vi "Initialize Data Channels.vi"(8 "error in (no error)":errorcluster, 10 "Framework Configuration":refnum<class "Framework Configuration.lvclass">, 11 "VeriStand Data Sharing Framework in":refnum<class "VeriStand DSF.lvclass">) -> (0 "error out":errorcluster, 1 "data channels refs":T1[](array[typedef]) format="%.0x", 2 "data channel offsets":u64[](array[numeric]) format="%.0x", 3 "VeriStand Data Sharing Framework out":refnum<class "VeriStand DSF.lvclass">)   [LabVIEW 2020, in "DSF Engine.lvlib" / "VeriStand DSF.lvclass"]
uses:
  VeriStand DSF.lvclass
  DSF Core.lvlibp/Classes/Configuration/Core/Framework/Framework Configuration.lvclass
  <vilib>/NI VeriStand/Custom Device API/Custom Device Item Ref.ctl
  VeriStand DSF.lvclass/VeriStand DSF.ctl
  <vilib>/NI VeriStand/Custom Device API/Data Access Type.ctl
  DSF Core.lvlibp/Typedefs/DSF Direction.ctl
  Data Channel Page GUID.vi
  <vilib>/NI VeriStand/Custom Device API/Custom Device API.lvlib
  Source/DSF Core.lvlibp
  DSF Shared.lvlib
  DSF Core.lvlibp/Classes/Configuration/Core/Thread/Thread Configuration.lvclass
  DSF Core.lvlibp/Classes/Configuration/Core/Plugin/Plugin Configuration.lvclass
  DSF Core.lvlibp/Classes/Configuration/Core/Group/Group Configuration.lvclass
  DSF Core.lvlibp/Classes/Configuration/Core/Transfer/Transfer Configuration.lvclass
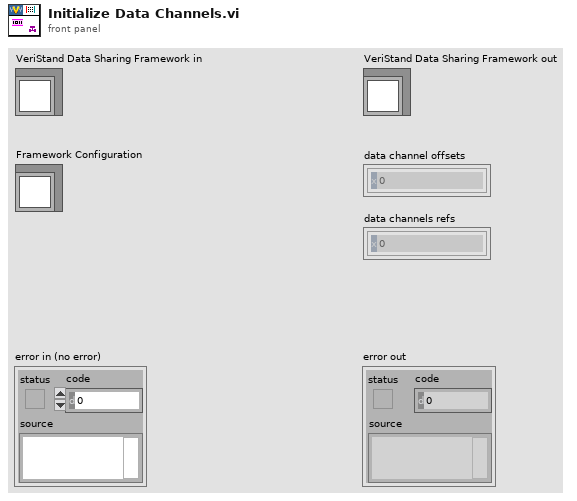
[diagram p1: front panel]
types:
  T1 = typedef "Custom Device API.lvlib/Custom Device Item Ref.ctl" = u64
  T2 = typedef "Custom Device API.lvlib/Data Access Type.ctl" = enum16{"Read", "Write"}
  T3 = typedef "DSF Core.lvlibp/DSF Direction.ctl" = enum8{"Tx", "Rx"}
  T4 = typedef "DSF Core.lvlibp/Group Configuration.lvclass/Core Group Configuration.ctl" = cluster{"name":string, "direction":T3, "cycle timing":T5, "timeout behavior":T6, "enable conversion":bool}
  T5 = typedef "DSF Core.lvlibp/DSF Timing Info.ctl" = cluster{"priority":u64, "decimation":u64, "offset":u64}
  T6 = typedef "DSF Core.lvlibp/DSF Timeout Behavior.ctl" = enum8{"Increment Late Count", "Throw Error"}
  T7 = typedef "DSF Core.lvlibp/Transfer Configuration.lvclass/Channel Configuration.ctl" = cluster{"configuration":T8, "component settings":T10[]}
  T8 = typedef "DSF Core.lvlibp/Channel Configuration.lvclass/Core Channel Configuration.ctl" = cluster{"name":string, "units":string, "engine data type":T9, "string data type":T9, "string offset":u64}
  T9 = typedef "DSF Core.lvlibp/DSF Data Type.ctl" = enum8{"Bool", "SGL", "DBL", "I8", "I16", "I32", "I64", "U8", "U16", "U32", "U64"}
  T10 = typedef "DSF Core.lvlibp/DSF Settings Info.ctl" = cluster{"component":string, "values":cluster{"key":string, "value":string}[]}
  T11 = typedef "Custom Device API.lvlib/Data Reference.ctl" = i32
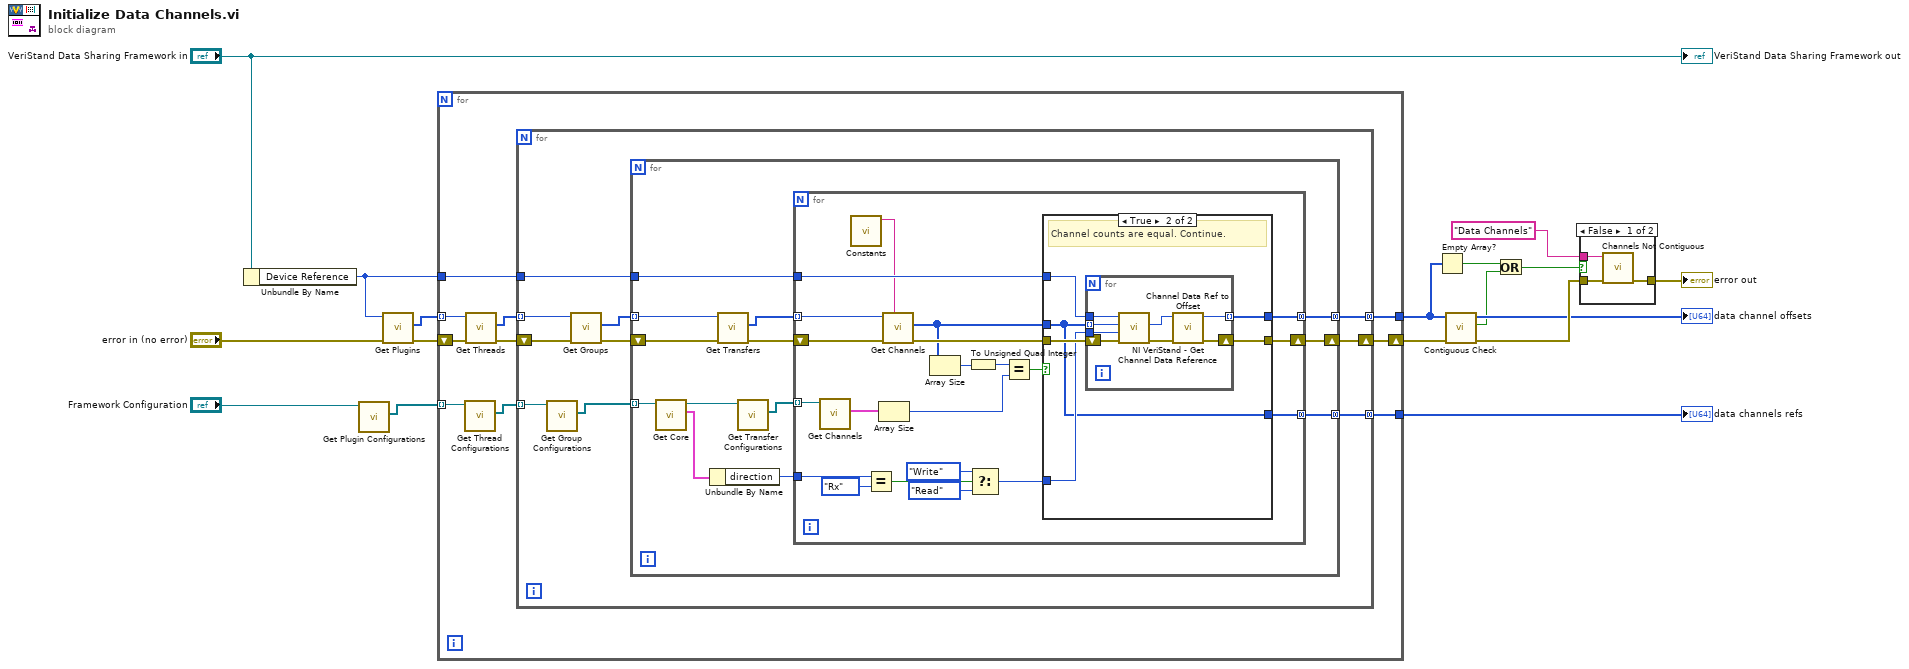
[diagram p0: block diagram]
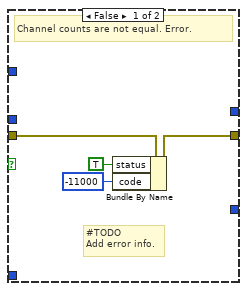
[diagram p2: hidden frame]
diagram:
  n1 = Unbundle By Name("VeriStand Data Sharing Framework in") -> ("Device Reference"=w13:T1)
  n2 = call "Get Plugin Configurations.vi"("Framework Configuration in"="Framework Configuration") -> ("Plugin Configurations"=w3:refnum<class "Plugin Configuration.lvclass">[])  [unwired: 8 in, 2 out]
  n3 = call "Get Plugins.vi"("error in (no error)"="error in (no error)", "Item Ref in"=w13) -> ("error out"=w16:errorcluster, "Plugin refs"=w15:T1[])  [unwired: 7 in, 1 out]
  n4 = for {
    tunnel: w15 -> [w22] mode=indexing
    tunnel: w13 -> [w26]
    tunnel: [w25] -> w10
    tunnel: [w24] -> w9
    tunnel: w3 -> [w19] mode=indexing
    shift-right: [w27] -> w17
    shift-left: w16 -> [w23]
    n5 = call "Get Thread Configurations.vi"("Plugin Configuration in"=w19) -> ("Thread Configurations"=w18:refnum<class "Thread Configuration.lvclass">[])  [unwired: 8 in, 2 out]
    n6 = call "Get Threads.vi"("error in (no error)"=w23, "Item Ref in"=w22) -> ("error out"=w21:errorcluster, "Plugin refs"=w20:T1[])  [unwired: 7 in, 1 out]
    n7 = for {
      tunnel: w20 -> [w33] mode=indexing
      tunnel: w18 -> [w29] mode=indexing
      tunnel: w26 -> [w37]
      shift-right: [w36] -> w27
      shift-left: w21 -> [w34]
      tunnel: [w35] -> w24 mode=concatenating
      tunnel: [w30] -> w25 mode=concatenating
      n8 = call "Get Group Configurations.vi"("Thread Configuration in"=w29) -> ("Group Configurations"=w28:refnum<class "Group Configuration.lvclass">[])  [unwired: 8 in, 2 out]
      n9 = call "Get Groups.vi"("error in (no error)"=w34, "Plugin Ref in"=w33) -> ("error out"=w32:errorcluster, "Group refs"=w31:T1[])  [unwired: 7 in, 1 out]
      n10 = for {
        tunnel: w28 -> [w42] mode=indexing
        tunnel: w31 -> [w46] mode=indexing
        tunnel: w37 -> [w50]
        shift-right: [w49] -> w36
        shift-left: w32 -> [w47]
        tunnel: [w48] -> w35 mode=concatenating
        tunnel: [w43] -> w30 mode=concatenating
        n11 = call "Get Core.vi"("Group Configuration in"=w42) -> ("core"=w38:T4, "Group Configuration out"=w41:refnum<class "Group Configuration.lvclass">)  [unwired: 8 in, 1 out]
        n12 = Unbundle By Name(w38) -> ("direction"=w39:T3)
        n13 = call "Get Transfers.vi"("error in (no error)"=w47, "Group Ref in"=w46) -> ("error out"=w45:errorcluster, "Transfer refs"=w44:T1[])  [unwired: 7 in, 1 out]
        n14 = call "Get Transfer Configurations.vi"("Group Configuration in"=w41) -> ("Transfer Configurations"=w40:refnum<class "Transfer Configuration.lvclass">[])  [unwired: 8 in, 2 out]
        n15 = for {
          tunnel: w40 -> [w53] mode=indexing
          tunnel: w44 -> [w60] mode=indexing
          tunnel: w50 -> [w64]
          shift-right: [w62] -> w49
          shift-left: w45 -> [w54]
          tunnel: [w61] -> w48 mode=concatenating
          tunnel: [w57] -> w43 mode=concatenating
          tunnel: w39 -> [w55]
          n16 = call "Get Channels.vi"("Transfer Configuration in"=w53) -> ("channels"=w52:T7[])  [unwired: 8 in, 2 out]
          n17 = call-poly "Constants.vi"() -> ("Status GUID"=w56:string)  [unwired: 11 in]
          n18 = Equal?(x=w55, y=DSF_Direction."Rx") -> (x = y?=w69:bool)
          n19 = Array Size(array=w52) -> (size(s)=w51:i32)
          n20 = call "Get Channels.vi"("GUID (Default Channel)"=w56, "error in (no error)"=w54, "Item Ref in"=w60) -> ("error out"=w59:errorcluster, "Channels refs"=w58:T1[])  [unwired: 6 in, 1 out]
          n21 = Array Size(array=w58) -> (size(s)=w71:i32)
          n22 = To Unsigned Quad Integer(1:w71) -> (0:w65:u64)
          n23 = Select(t=Data_Access_Type."Write" ("Access"), s=w69, f=Data_Access_Type."Read") -> (s? t:f=w63:T2)
          n24 = Equal?(x=w65, y=w51) -> (x = y?=w66:bool)
          n25 = case shown="True" w66 {
            tunnel: w58 -> [_ w76]
            tunnel: w64 -> [_ w80]
            tunnel: w63 -> [_ w79]
            tunnel: w59 -> [w75 w81]
            tunnel: [w74 w77] -> w62
            tunnel: [_ w78] -> w61
            tunnel: [_ w76] -> w57
            frame False {
              # "#TODO\nAdd error info."
              # "Channel counts are not equal. Error."
              n26 = Bundle By Name(cluster=w75, "status"=TRUE, "code"=-11000) -> (w74:errorcluster)
            }
            frame True {
              # "Channel counts are equal. Continue."
              n27 = for {
                tunnel: w80 -> [w88]
                tunnel: w79 -> [w87]
                tunnel: w76 -> [w86] mode=indexing
                tunnel: [w82] -> w78 mode=indexing
                shift-right: [w83] -> w77
                shift-left: w81 -> [w89]
                n28 = call <vilib>:"NI VeriStand - Get Channel Data Reference.vi"("error in (no error)"=w89, "Access"=w87, "Channel Ref in"=w86, "Device Ref in"=w88) -> ("error out"=w85:errorcluster, "Channel Data Reference"=w84:T11)  [unwired: 5 in, 1 out]
                n29 = call "Channel Data Ref to Offset.vi"("error in (no error)"=w85, "Channel Data Reference"=w84) -> ("error out"=w83:errorcluster, "channel offset"=w82:u64)  [unwired: 8 in]
              }
            }
          }
        }
      }
    }
  }
  "data channels refs" <- w10
  n30 = Empty Array?(array=w9) -> (empty?=w8:bool)
  n31 = call "Contiguous Check.vi"("error in (no error)"=w17, "channel offsets in"=w9) -> ("error out"=w12:errorcluster, "contiguous?"=w5:bool, "channel offsets out"=→"data channel offsets":u64[])  [unwired: 7 in]
  n32 = Or(x=w8, y=w5) -> (x .or. y?=w7:bool)
  n33 = case shown="False" w7 {
    tunnel: [w92 w93] -> w11
    tunnel: w12 -> [w91 w93]
    tunnel: "Data Channels" ("name") -> [w90 _]
    frame False {
      n34 = call "Channels Not Contiguous.vi"("error in (no error)"=w91, "name"=w90) -> ("error out"=w92:errorcluster)  [unwired: 9 in]
    }
    frame True {
    }
  }
  "error out" <- w11
  "VeriStand Data Sharing Framework out" <- "VeriStand Data Sharing Framework in"
